vi "LockIntoSignal.vi"(10 "GPIB Address":string, 11 "error in":errorcluster) -> (0 "error out":errorcluster)   [LabVIEW 2017, in "LD Reading.lvclass"]
uses:
  LD Reading.lvclass
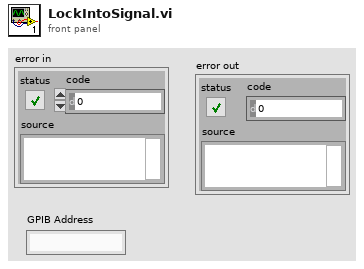
[diagram p1: front panel]
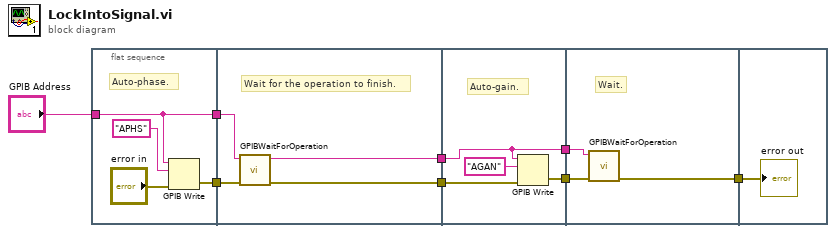
[diagram p0: block diagram]
diagram:
  n1 = flat-sequence {
    tunnel: [w11] -> w7
    tunnel: "GPIB Address" -> [w9]
    tunnel: [w9] -> w6
    tunnel: w6 -> [w16]
    tunnel: w7 -> [w14]
    tunnel: [w15] -> w5
    tunnel: [w13] -> w4
    tunnel: w5 -> [w19]
    tunnel: w4 -> [w18]
    tunnel: [w18] -> w3
    tunnel: [w17] -> w2
    tunnel: w3 -> [w23]
    tunnel: w2 -> [w22]
    tunnel: [w21] -> w1
    tunnel: w1 -> [w24]
    frame #0 {
      # "Auto-phase."
      n2 = GPIB Write(0:w9, 1:"APHS" ("data"), 3:"error in") -> (6:w11:errorcluster)  [unwired: 2 in, 1 out]
    }
    frame #1 {
      # "Wait for the operation to finish."
      n3 = call "GPIBWaitForOperation.vi"("error in (no error)"=w14, "GPIB Address in"=w16) -> ("error out"=w15:errorcluster, "GPIB Address out"=w13:string)  [unwired: 8 in]
    }
    frame #2 {
      # "Auto-gain."
      n4 = GPIB Write(0:w18, 1:"AGAN" ("data"), 3:w19) -> (6:w17:errorcluster)  [unwired: 2 in, 1 out]
    }
    frame #3 {
      # "Wait."
      n5 = call "GPIBWaitForOperation.vi"("error in (no error)"=w22, "GPIB Address in"=w23) -> ("error out"=w21:errorcluster)  [unwired: 8 in, 1 out]
    }
    frame #4 {
      "error out" <- w24
    }
  }
